vi "DetectorGlobals.vi"() -> ()   [LabVIEW 2014]
panel:
  out "NumFT":i32=1
  out "DarkRows":i32=1
  out "DarkCols":i32=1
  out "DevRows":i32=1
  out "DevCols":i32=1
  out "AmpConfig":string
  out "SetTemperature":dbl
  out "Gain":i32=2
  out "Amp":i32
  out "OverRows":i32
  out "UnderRows":i32
  out "OverCols":i32=20
  out "UnderCols":i32
  out "LastRow":i32=4064
  out "FirstRow":i32=1
  out "LastCol":i32=4064
  out "FirstCol":i32=1
  out "ColBin":i32=1
  out "RowBin":i32=1
  # "Video"
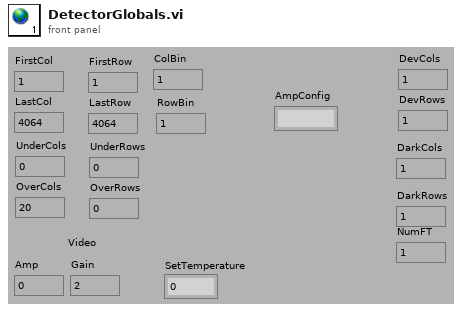
[diagram p1: front panel]
diagram:
